vi "DeviceClose.vi"(6 "Delay between send and receive [ms]":i32=100, 8 "error in (no error)":errorcluster, 11 "GenericDevice in":refnum<class "GenericDevice.lvclass">) -> (0 "error out":errorcluster, 1 "ID":i32, 2 "results-JSON string":string, 3 "GenericDevice out":refnum<class "GenericDevice.lvclass">, 4 "device is open?":bool)   [LabVIEW 2023, in "GenericDevice.lvclass"]
doc: "Closes communications with the CCD indicated by the index."
uses:
  GenericDevice.lvclass
  GenericDevice.lvclass/GenericDevice.ctl
  53f75d40-961b-4401-a988-894ae3dfba8f.vi
  b3af86d2-a35b-4918-bc34-7d490bf60e23.vi
  <vilib>/JDP Science/JSONtext/Variant to JSON Text.vi
  <vilib>/JDP Science/JSONtext/Set Item.vi
  <vilib>/JDP Science/JSONtext/LVClass Serializer/JSONtext LVClass Serializer.lvclass
panel:
  # "Connector Pane"
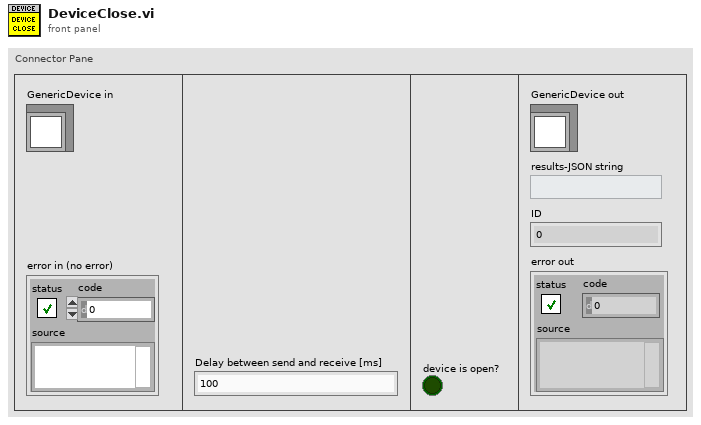
[diagram p1: front panel]
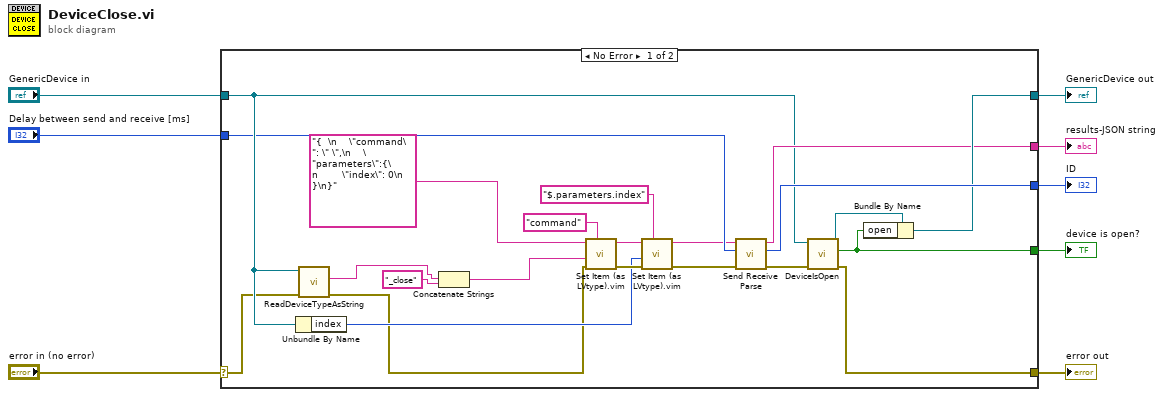
[diagram p0: block diagram]
diagram:
  n1 = case shown="No Error" "error in (no error)" {
    selector: "error in (no error)" -> [w12 w32]
    tunnel: [w17 w32] -> w7
    tunnel: [w19 w31] -> w5
    tunnel: "GenericDevice in" -> [w14 w31]
    tunnel: [w22 _] -> w4
    tunnel: [w16 _] -> w3
    tunnel: [w15 _] -> w2
    tunnel: "Delay between send and receive [ms]" -> [w10 _]
    frame No Error {
      n2 = Unbundle By Name(w14) -> ("index"=w23:i32)
      n3 = call "ReadDeviceTypeAsString.vi"("error in (no error)"=w12, "GenericDevice.lvclass"=w14) -> ("error out"=w11:errorcluster, "String"=w13:string)  [unwired: 7 in, 1 out]
      n4 = Concatenate Strings(w13, "_close" ("string")) -> (w24:string)
      n5 = call "Set Item (as LVtype).vim"("$Path or Item Name"="command", "error in (no error)"=w11, "Anything"=w24, "JSON"="{  \n    \"command\": \" \",\n    \"parameters\":{\n        \"index\": 0\n    }\n}") -> ("error out"=w28:errorcluster, "<JSON>"=w29:string)  [unwired: 4 in, 1 out]
      n6 = call "Set Item (as LVtype).vim"("$Path or Item Name"="$.parameters.index", "error in (no error)"=w28, "Anything"=w23, "JSON"=w29) -> ("error out"=w21:errorcluster, "<JSON>"=w9:string)  [unwired: 4 in, 1 out]
      n7 = call "Send Receive Parse.vi"("error in"=w21, "Delay between send and receive [ms]"=w10, "<JSON>"=w9) -> ("error out"=w18:errorcluster, "ID"=w22:i32, "results-JSON string"=w15:string)  [unwired: 6 in]
      n8 = call-dynamic "DeviceIsOpen.vi"("error in (no error)"=w18, "GenericDevice in"=w14) -> ("error out"=w17:errorcluster, "device is open?"=w16:bool, "GenericDevice out"=w20:refnum<class "GenericDevice.lvclass">)  [unwired: 6 in, 1 out]
      n9 = Bundle By Name(cluster=w20, "open"=w16) -> (w19:refnum<class "GenericDevice.lvclass">)
    }
    frame Error {
    }
  }
  "error out" <- w7
  "GenericDevice out" <- w5
  "ID" <- w4
  "device is open?" <- w3
  "results-JSON string" <- w2
